vi "Set Local Variables.vi"(6 "Local Variable Top Level":string, 8 "error in (no error)":errorcluster, 9 "Local Variable Mapping":string[](array[string]), 10 "Values(As String)":string[](array[string]), 11 "QPA Measurement In":refnum<class "QPA Measurement.lvclass">) -> (0 "error out":errorcluster, 3 "QPA Measurement Out":refnum<class "QPA Measurement.lvclass">)   [LabVIEW 2016, in "QPA Measurement.lvlib" / "QPA Measurement.lvclass"]
uses:
  QPA Measurement.lvclass
  QPA Measurement.lvclass/QPA Measurement.ctl
  Read Sequence Reference.vi
  Plugins/TestStand API Tools (TSAT).lvlibp/Sequence Actions/TSAT Sequence Actions.lvlib
  Plugins/TestStand API Tools (TSAT).lvlibp/TSAT Utilities/TSAT Utilities.lvlib
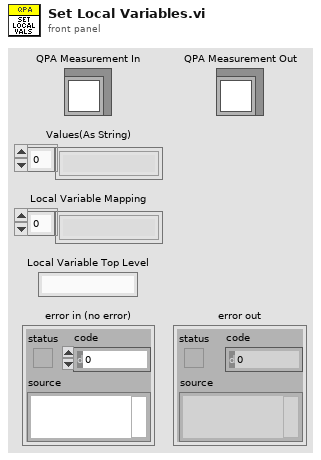
[diagram p1: front panel]
types:
  T1 = enum16{"Container", "String", "Boolean", "Number", "NamedType", "Reference", "Array"}
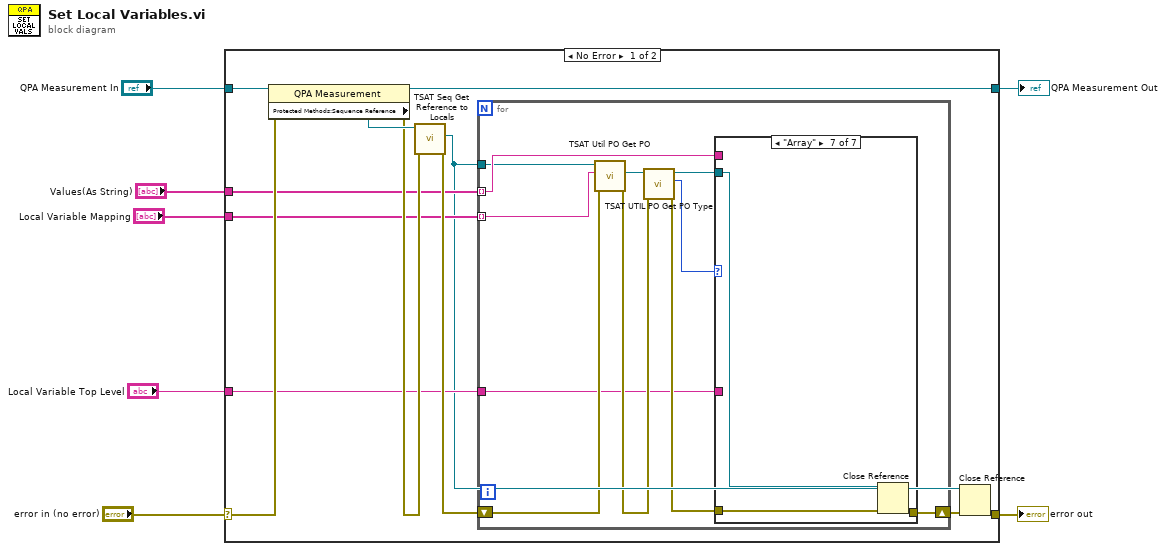
[diagram p0: block diagram]
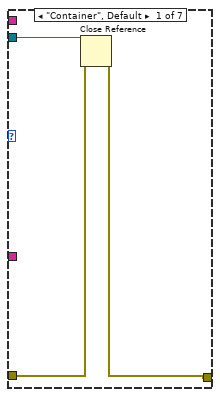
[diagram p2: hidden frame]
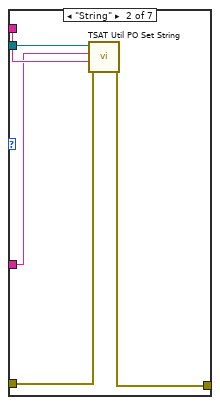
[diagram p3: hidden frame]
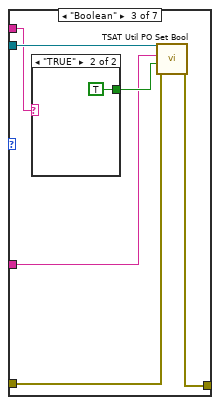
[diagram p4: hidden frame]
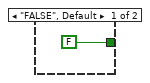
[diagram p5: hidden frame]
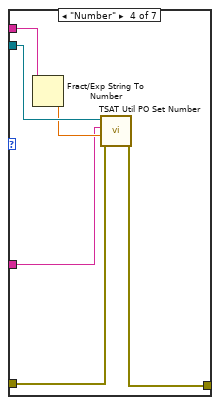
[diagram p6: hidden frame]
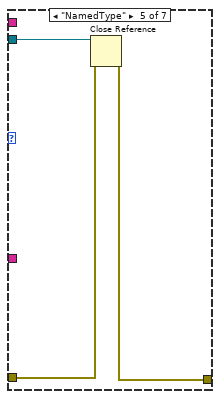
[diagram p7: hidden frame]
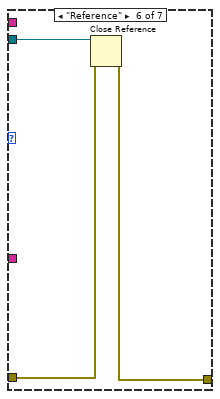
[diagram p8: hidden frame]
diagram:
  n1 = case shown="No Error" "error in (no error)" {
    selector: "error in (no error)" -> [w19 w63]
    tunnel: [w9 w63] -> w6
    tunnel: [w17 w62] -> w4
    tunnel: "QPA Measurement In" -> [w18 w62]
    tunnel: "Values(As String)" -> [w13 _]
    tunnel: "Local Variable Mapping" -> [w12 _]
    tunnel: "Local Variable Top Level" -> [w10 _]
    frame No Error {
      n2 = property class="QPA Measurement"(reference=w18, error in=w19) -> (reference out=w17:refnum<class "QPA Measurement.lvclass">, error out=w15:errorcluster, "Protected Methods:Sequence Reference"=w16:refnum<k7>)
      n3 = call "TSAT Seq Get Reference to Locals.vi"("Error In"=w15, "Sequence In"=w16) -> ("Error Out"=w14:errorcluster, "Locals"=w8:refnum<k7>)  [unwired: 7 in, 1 out]
      n4 = for {
        tunnel: w8 -> [w29]
        tunnel: w13 -> [w30] mode=indexing
        tunnel: w12 -> [w28] mode=indexing
        shift-right: [w21] -> w11
        shift-left: w14 -> [w24]
        tunnel: w10 -> [w20]
        n5 = call "TSAT Util PO Get PO.vi"("error in (no error)"=w24, "Sub Property to Retrieve"=w28, "Property Object in"=w29) -> ("error out"=w23:errorcluster, "SubProperty"=w27:refnum<k7>)  [unwired: 6 in, 1 out]
        n6 = call "TSAT UTIL PO Get PO Type.vi"("error in (no error)"=w23, "PropertyObject In"=w27) -> ("error out"=w22:errorcluster, "PropertyObject Type"=w25:T1, "PropertyObject Out"=w26:refnum<k7>)  [unwired: 7 in]
        n7 = case shown="\"Array\"" w25 {
          tunnel: w26 -> [w33 w38 w44 w52 w55 w58 w61]
          tunnel: w30 -> [_ w37 w41 w49 _ _ _]
          tunnel: w22 -> [w32 w36 w43 w51 w54 w57 w60]
          tunnel: [w31 w35 w42 w50 w53 w56 w59] -> w21
          tunnel: w20 -> [_ w34 w39 w47 _ _ _]
          frame "Container", Default {
            n8 = Close Reference(reference=w33, error in (no error)=w32) -> (error out=w31:errorcluster)
          }
          frame "String" {
            n9 = call "TSAT Util PO Set String.vi"("error in (no error)"=w36, "Variable Value"=w37, "Local Variable Name"=w34, "Property Object in"=w38) -> ("error out"=w35:errorcluster)  [unwired: 7 in]
          }
          frame "Boolean" {
            n10 = case shown="\"TRUE\"" w41 {
              tunnel: [FALSE TRUE] -> w40
              frame "FALSE", Default {
              }
              frame "TRUE" {
              }
            }
            n11 = call "TSAT Util PO Set Bool.vi"("error in (no error)"=w43, "Variable Value"=w40, "Local Variable Name"=w39, "Property Object in"=w44) -> ("error out"=w42:errorcluster)  [unwired: 7 in]
          }
          frame "Number" {
            n12 = Fract/Exp String To Number(string=w49) -> (number=w48:dbl)  [unwired: 3 in, 1 out]
            n13 = call "TSAT Util PO Set Number.vi"("error in (no error)"=w51, "Variable Value"=w48, "Local Variable Name"=w47, "Property Object in"=w52) -> ("error out"=w50:errorcluster)  [unwired: 7 in]
          }
          frame "NamedType" {
            n14 = Close Reference(reference=w55, error in (no error)=w54) -> (error out=w53:errorcluster)
          }
          frame "Reference" {
            n15 = Close Reference(reference=w58, error in (no error)=w57) -> (error out=w56:errorcluster)
          }
          frame "Array" {
            n16 = Close Reference(reference=w61, error in (no error)=w60) -> (error out=w59:errorcluster)
          }
        }
      }
      n17 = Close Reference(reference=w8, error in (no error)=w11) -> (error out=w9:errorcluster)
    }
    frame Error {
    }
  }
  "error out" <- w6
  "QPA Measurement Out" <- w4
